vi "Write.vi"(8 "Error In":errorcluster, 10 "Content":string, 11 "Writer In":refnum<class "Abstract.lvclass">) -> (0 "Error Out":errorcluster, 3 "Writer Out":refnum<class "Abstract.lvclass">)   [LabVIEW 2018, in "Toolkit.lvlib" / "Writers.lvlib" / "Abstract.lvclass"]
doc: "Writes a rendered Mustache template to a destination."
uses:
  Abstract.lvclass
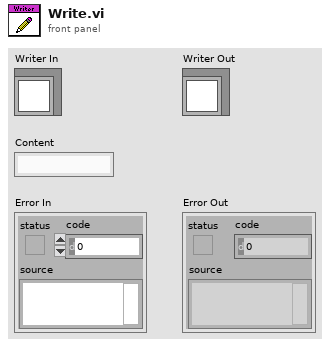
[diagram p1: front panel]
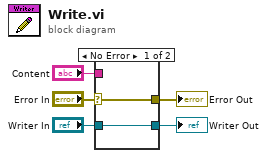
[diagram p0: block diagram]
diagram:
  n1 = case shown="No Error" "Error In" {
    selector: "Error In" -> [w6 w9]
    tunnel: [w6 w9] -> w4
    tunnel: [w7 w8] -> w2
    tunnel: "Writer In" -> [w7 w8]
    tunnel: "Content" -> [_ _]
    frame No Error {
    }
    frame Error {
    }
  }
  "Error Out" <- w4
  "Writer Out" <- w2
